vi "ROI group interface-Find POI within group boundaries.vi"(8 "error in (no error)":errorcluster, 9 "X-Y coordinates array of POI":i64[][](array[numeric]), 10 "ROI Descriptor Out":T2 {"Contours"."Type" items=["No Selection", "Point", "Line", "Rectangle", "Oval", "Polygon", "Freehand Region", "Annulus", "Unused2", "Unused3", "Broken Line", "Freehand Line", "Rotated Rectangle"]}, 11 "Image ref in":T1) -> (0 "error out":errorcluster, 1 "# of POI in group":i32, 2 "ROI to be grouped":i32[](array[numeric]), 3 "Image ref shift out":T1)   [LabVIEW 2013]
uses:
  <vilib>/vision/Image Controls.llb/IMAQ Image.ctl
  <vilib>/vision/NI_Vision_Development_Module.lvlib
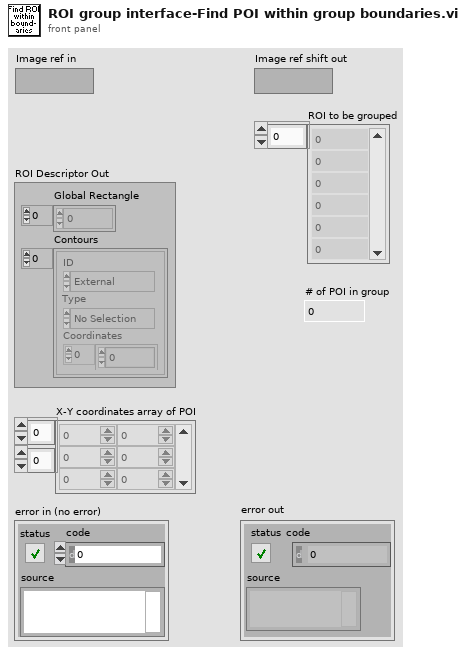
[diagram p1: front panel]
types:
  T1 = typedef "IMAQ Image.ctl" = refnum<image>
  T2 = typedef "ROI Descriptor" = cluster{"Global Rectangle":i32[], "Contours":cluster{"ID":enum32{"External", "Internal"}, "Type":u32, "Coordinates":i32[]}[]}
  T3 = typedef "IMAQ Point" = cluster{"X":sgl, "Y":sgl}
  T4 = typedef "Image Type" = u32
  T5 = cluster{"histogram":u32[], "Minimal Value":sgl, "Maximal Value":sgl, "Starting Value":sgl, "Interval Width":sgl, "Mean Value":sgl, "Standard  Variation":sgl, "Area (pixels)":i32}
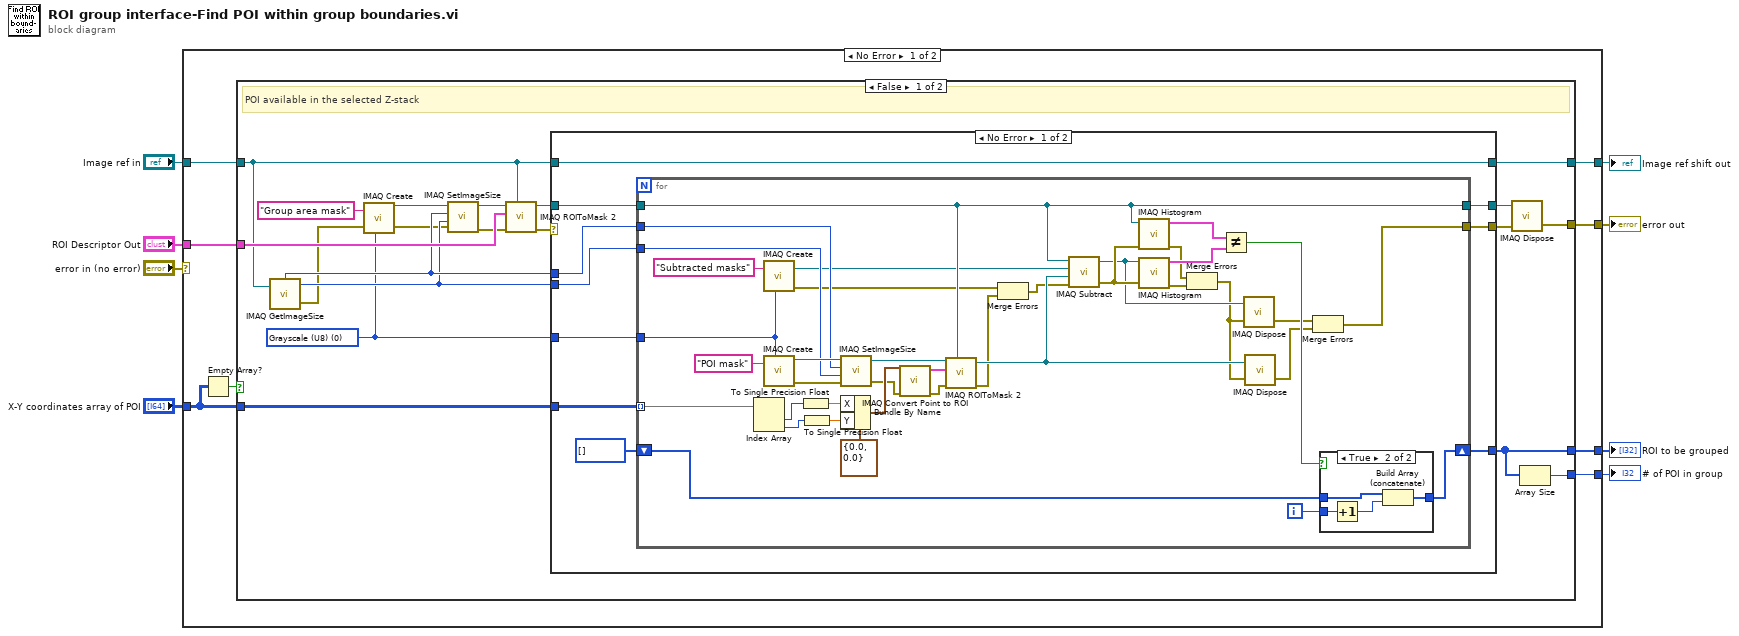
[diagram p0: block diagram]
diagram:
  n1 = case shown="No Error" "error in (no error)" {
    selector: "error in (no error)" -> [_ w95]
    tunnel: [w16 _] -> w8
    tunnel: [w15 _] -> w7
    tunnel: "ROI Descriptor Out" -> [w14 _]
    tunnel: "Image ref in" -> [w13 w94]
    tunnel: [w12 w95] -> w5
    tunnel: "X-Y coordinates array of POI" -> [w10 _]
    tunnel: [w9 w94] -> w2
    frame No Error {
      n2 = Empty Array?(array=w10) -> (empty?=w11:bool)
      n3 = case shown="False" w11 {
        tunnel: [w32 _] -> w16
        tunnel: [w31 _] -> w15
        tunnel: w14 -> [w30 _]
        tunnel: w13 -> [w18 w93]
        tunnel: [w26 _] -> w12
        tunnel: w10 -> [w25 _]
        tunnel: [w24 w93] -> w9
        frame False {
          w17 = T4 0 items=["Grayscale (U8)", "Grayscale (I16)", "Grayscale (SGL)", "Complex (CSG)", "RGB (U32)", "HSL (U32)", "RGB (U64)", "Grayscale (U16)"] ("Image Type")
          # "POI available in the selected Z-stack"
          n4 = call "IMAQ GetImageSize"("Image"=w18) -> ("Y Resolution"=w22:i32, "X Resolution"=w23:i32, "error out"=w20:errorcluster)  [unwired: 3 in]
          n5 = call "IMAQ Create"("Image Name"="Group area mask" ("string"), "Image Type"=w17, "error in (no error)"=w20) -> ("New Image"=w35:T1, "error out"=w21:errorcluster)  [unwired: 2 in]
          n6 = call "IMAQ SetImageSize"("error in (no error)"=w21, "Y Resolution"=w22, "X Resolution"=w23, "Image"=w35) -> ("error out"=w29:errorcluster, "Image Out"=w19:T1)  [unwired: 1 in]
          n7 = call "IMAQ ROIToMask 2"("Image Model"=w18, "error in (no error)"=w29, "ROI Descriptor"=w30, "Image"=w19) -> ("error out"=w28:errorcluster, "Image Out"=w33:T1)  [unwired: 5 in, 1 out]
          n8 = case shown="No Error" w28 {
            selector: w28 -> [_ w92]
            tunnel: [w46 w91] -> w36
            tunnel: w33 -> [w45 w91]
            tunnel: [w44 _] -> w31
            tunnel: w25 -> [w42 _]
            tunnel: w18 -> [w40 w90]
            tunnel: [w43 w92] -> w27
            tunnel: [w40 w90] -> w24
            tunnel: w23 -> [w39 _]
            tunnel: w22 -> [w38 _]
            tunnel: w17 -> [w37 _]
            frame No Error {
              n9 = for {
                tunnel: w45 -> [w56]
                tunnel: w42 -> [w80] mode=indexing
                shift-right: [w68] -> w44
                shift-left: i32[] [] -> [w67]
                tunnel: [w56] -> w46
                tunnel: [w63] -> w43
                tunnel: w39 -> [w61]
                tunnel: w38 -> [w60]
                tunnel: w37 -> [w59]
                i -> [w69]
                n10 = Index Array(array=w80) -> (element #1=w79:i64, element #2=w78:i64)  [unwired: 2 in]
                n11 = call "IMAQ Create"("Image Name"="Subtracted masks" ("string"), "Image Type"=w59) -> ("New Image"=w53:T1, "error out"=w52:errorcluster)  [unwired: 3 in]
                n12 = call "IMAQ Create"("Image Name"="POI mask" ("string"), "Image Type"=w59) -> ("New Image"=w75:T1, "error out"=w66:errorcluster)  [unwired: 3 in]
                n13 = To Single Precision Float(number=w79) -> (single precision float=w55:sgl)
                n14 = To Single Precision Float(number=w78) -> (single precision float=w54:sgl)
                n15 = call "IMAQ SetImageSize"("error in (no error)"=w66, "Y Resolution"=w60, "X Resolution"=w61, "Image"=w75) -> ("error out"=w48:errorcluster, "Image Out"=w58:T1)  [unwired: 1 in]
                n16 = Bundle By Name(cluster=T3 {"X"=0.0, "Y"=0.0} ("Point"), "X"=w55, "Y"=w54) -> (w77:T3)
                n17 = call "IMAQ Convert Point to ROI"("error in (no error)"=w48, "Point"=w77) -> ("error out"=w47:errorcluster, "ROI Descriptor"=w84:T2)  [unwired: 7 in]
                n18 = call "IMAQ ROIToMask 2"("Image Model"=w56, "error in (no error)"=w47, "ROI Descriptor"=w84, "Image"=w58) -> ("error out"=w51:errorcluster, "Image Out"=w62:T1)  [unwired: 5 in, 1 out]
                n19 = Merge Errors(w52, w51) -> (w50:errorcluster)
                n20 = call "IMAQ Subtract"("Image Src A"=w56, "Image Dst"=w53, "Image Src B"=w62, "error in (no error)"=w50) -> ("Image Dst Out"=w57:T1, "error out"=w73:errorcluster)  [unwired: 3 in]
                n21 = call "IMAQ Histogram"("error in (no error)"=w73, "Image"=w56) -> ("error out"=w72:errorcluster, "Histogram Report"=w83:T5)  [unwired: 8 in]
                n22 = call "IMAQ Histogram"("error in (no error)"=w73, "Image"=w57) -> ("error out"=w71:errorcluster, "Histogram Report"=w82:T5)  [unwired: 8 in]
                n23 = Merge Errors(w72, w71) -> (w49:errorcluster)
                n24 = Not Equal?(x=w83, y=w82) -> (x != y?=w70:bool)
                n25 = call "IMAQ Dispose"("Image"=w57, "error in (no error)"=w49) -> ("error out"=w65:errorcluster)  [unwired: 4 in]
                n26 = call "IMAQ Dispose"("Image"=w62, "error in (no error)"=w49) -> ("error out"=w64:errorcluster)  [unwired: 4 in]
                n27 = Merge Errors(w65, w64) -> (w63:errorcluster)
                n28 = case shown="True" w70 {
                  tunnel: w69 -> [_ w89]
                  tunnel: [w85 w88] -> w68
                  tunnel: w67 -> [w85 w87]
                  frame False {
                  }
                  frame True {
                    n29 = Increment(x=w89) -> (x+1=w86:i32)
                    n30 = Build Array (concatenate)(w87, w86) -> (w88:i32[])
                  }
                }
              }
            }
            frame Error {
            }
          }
          n31 = call "IMAQ Dispose"("Image"=w36, "error in (no error)"=w27) -> ("error out"=w26:errorcluster)  [unwired: 4 in]
          n32 = Array Size(array=w31) -> (size(s)=w32:i32)
        }
        frame True {
          # "No POI available in the selected Z-stack"
        }
      }
    }
    frame Error {
    }
  }
  "ROI to be grouped" <- w7
  "# of POI in group" <- w8
  "error out" <- w5
  "Image ref shift out" <- w2
